vi "Terminal Block.vi"(11 "Block":refnum<class "Block.lvclass">) -> ()   [LabVIEW 2020, in "Parallel Block.lvlib" / "Manager.lvclass"]
uses:
  Manager.lvclass
  Manager.lvclass/Manager.ctl
  Block/Block.lvclass
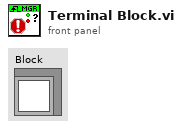
[diagram p1: front panel]
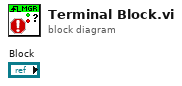
[diagram p0: block diagram]
diagram:
